vi "PM100D_SensorFlag.vi"(8 "error in (no error)":errorcluster, 11 "VISA in":refnum<visa-resource-name>) -> (0 "error out":errorcluster, 1 "flags":bool[](array[boolean]), 2 "cal_msg":string, 3 "VISA out":refnum<visa-resource-name>, 4 "subtype":i32, 5 "sn":string, 6 "type":i32, 7 "name":string)   [LabVIEW 2010]
doc: "This VI queries all relevant sensor info:\n- sensor name\n- sensor serial number\n- calibration message\n- sensor type\n- sensor sub-type\n- sensor flags"
panel:
  # "1 Power Sensor"
  # "2 Energy Sensor"
  # "4"
  # "8"
  # "16 Response settable"
  # "32 Wavelength settable"
  # "64 Tau (time constant) settable"
  # "128"
  # "256 With temperature sensor"
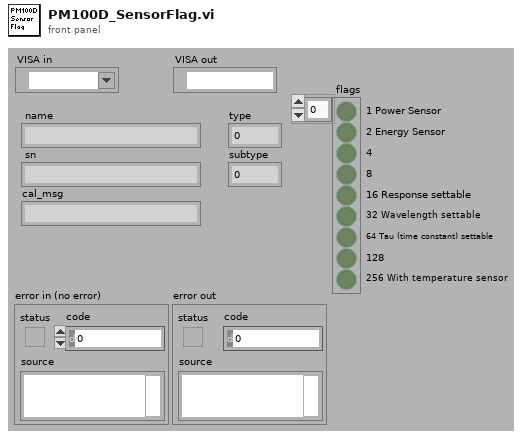
[diagram p1: front panel]
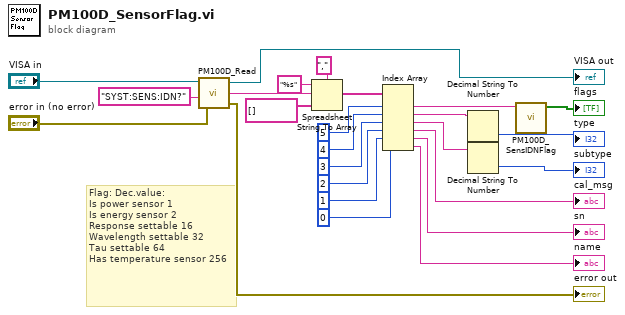
[diagram p0: block diagram]
diagram:
  # "Flag:\tDec.value:\nIs power sensor\t1\nIs energy sensor\t2\nResponse settable\t16\nWavelength settable\t32\nTau settable\t64\nHas temperature sensor\t256"
  n1 = call "PM100D_Read.vi"("error in (no error)"="error in (no error)", "Command"="SYST:SENS:IDN?", "VISA in"="VISA in") -> ("error out"=→"error out":errorcluster, "ReadValue"=w18:string, "VISA out"=→"VISA out":refnum<visa-resource-name>)  [unwired: 1 in]
  n2 = Spreadsheet String To Array(delimiter (Tab)=",", format string="%s", spreadsheet string=w18, array type (2D Dbl)=string[] [] ("Rng_Array")) -> (array=w20:string[])
  n3 = Index Array(array=w20, index #1=5 ("index"), index #2=4 ("index"), index #3=3 ("index"), index #4=2 ("index"), index #5=1 ("index"), index #6=0 ("index")) -> (element #1=w23:string, element #2=w3:string, element #3=w4:string, element #4=→"cal_msg":string, element #5=→"sn":string, element #6=→"name":string)
  n4 = Decimal String To Number(string=w3) -> (number=→"type":i32)  [unwired: 2 in, 1 out]
  n5 = Decimal String To Number(string=w4) -> (number=→"subtype":i32)  [unwired: 2 in, 1 out]
  n6 = call "PM100D_SensIDNFlag.vi"("String"=w23) -> ("Flag"=→"flags":bool[])  [unwired: 6 out]
